vi "loadSingleToneRampData.vi"(8 "error in (no error)":errorcluster, 10 "toneRamp":refnum<class "SingleToneRamp.lvclass">, 11 "SingleToneRampAction in":refnum<class "SingleToneRampAction.lvclass">) -> (0 "error out":errorcluster, 2 "toneRampOut":refnum<class "SingleToneRamp.lvclass">, 3 "SingleToneRampAction out":refnum<class "SingleToneRampAction.lvclass">)   [LabVIEW 2011, in "Views.lvlib" / "ScriptEditor.lvlib" / "SingleToneRampAction.lvclass"]
uses:
  SingleToneRampAction.lvclass
  Tools/Scripting/ScriptingEvent/ScriptEvents/SingleTone/SingleToneRamp/SingleToneRamp.lvclass
  SingleToneRampAction.lvclass/SingleToneRampAction.ctl
  Tools/Scripting/ScriptingEvent/ScriptEvents/SingleTone/SingleTone.lvclass
  Tools/Scripting/ScriptingEvent/ScriptEvent.lvclass
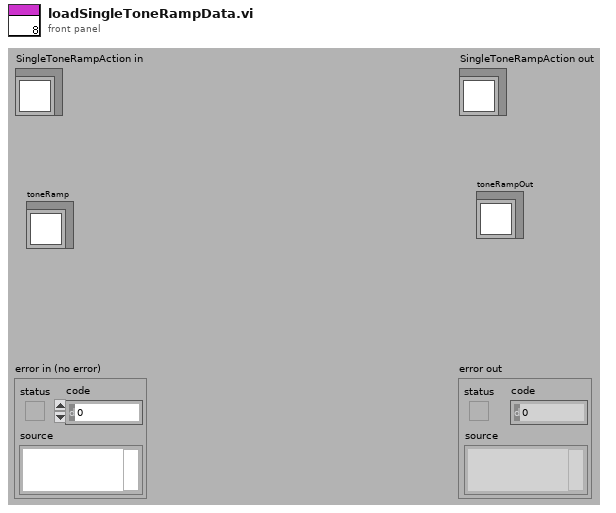
[diagram p1: front panel]
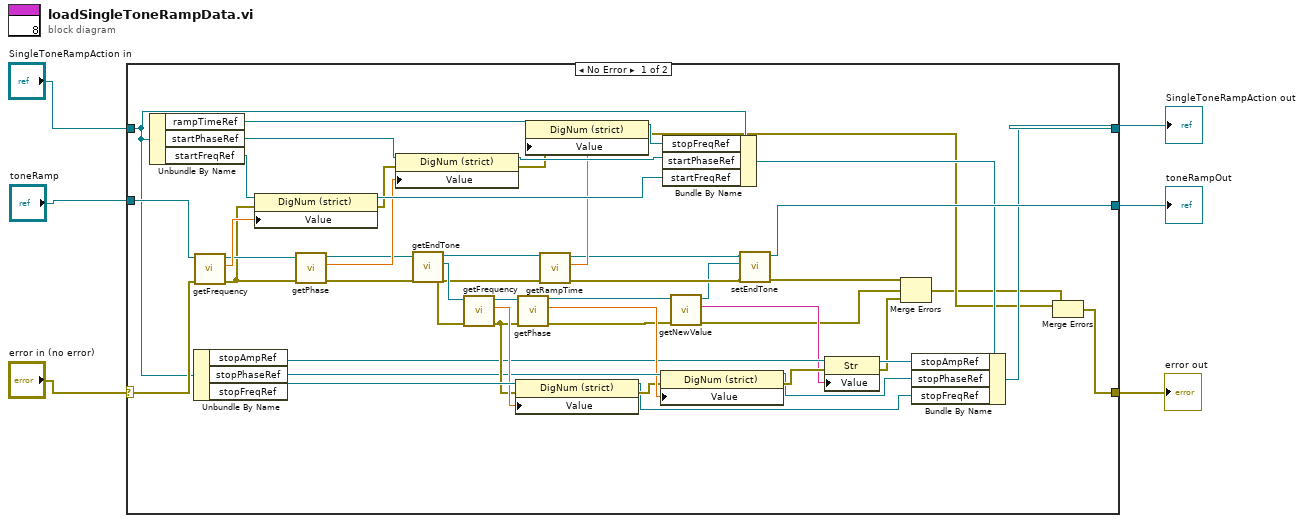
[diagram p0: block diagram]
diagram:
  n1 = case shown="No Error" "error in (no error)" {
    selector: "error in (no error)" -> [w54 w56]
    tunnel: [w12 w56] -> w2
    tunnel: [w13 w55] -> w3
    tunnel: "SingleToneRampAction in" -> [w38 w55]
    tunnel: "toneRamp" -> [w43 _]
    tunnel: [w18 _] -> w1
    frame No Error {
      n2 = Unbundle By Name(w38) -> ("rampTimeRef"=w46:refnum<vi>, "startPhaseRef"=w50:refnum<vi>, "startFreqRef"=w53:refnum<vi>)
      n3 = Unbundle By Name(w38) -> ("stopAmpRef"=w24:refnum<vi>, "stopPhaseRef"=w30:refnum<vi>, "stopFreqRef"=w37:refnum<vi>)
      n4 = call "getFrequency.vi"("error in (no error)"=w54, "SingleTone.lvclass in"=w43) -> ("error out"=w42:errorcluster, "frequency"=w52:dbl, "SingleTone.lvclass out"=w48:refnum<class "SingleToneRamp.lvclass">)  [unwired: 7 in]
      n5 = property class="DigNum (strict)"(reference=w53, error in=w42, "Value"=w52) -> (reference out=w51:refnum<vi>, error out=w41:errorcluster)
      n6 = call "getPhase.vi"("error in (no error)"=w42, "SingleTone.lvclass in"=w48) -> ("error out"=w35:errorcluster, "phase"=w44:dbl, "SingleTone.lvclass out"=w36:refnum<class "SingleToneRamp.lvclass">)  [unwired: 7 in]
      n7 = property class="DigNum (strict)"(reference=w50, error in=w41, "Value"=w44) -> (reference out=w49:refnum<vi>, error out=w47:errorcluster)
      n8 = call "getEndTone.vi"("error in (no error)"=w35, "SingleToneRamp.lvclass in"=w36) -> ("error out"=w33:errorcluster, "endTone"=w39:refnum<class "SingleTone.lvclass">, "SingleToneRamp.lvclass out"=w34:refnum<class "SingleToneRamp.lvclass">)  [unwired: 7 in]
      n9 = call "getFrequency.vi"("error in (no error)"=w33, "SingleTone.lvclass in"=w39) -> ("error out"=w31:errorcluster, "frequency"=w32:dbl, "SingleTone.lvclass out"=w28:refnum<class "SingleTone.lvclass">)  [unwired: 7 in]
      n10 = property class="DigNum (strict)"(reference=w37, error in=w31, "Value"=w32) -> (reference out=w15:refnum<vi>, error out=w25:errorcluster)
      n11 = call "getPhase.vi"("error in (no error)"=w31, "SingleTone.lvclass in"=w28) -> ("error out"=w26:errorcluster, "phase"=w29:dbl, "SingleTone.lvclass out"=w27:refnum<class "SingleTone.lvclass">)  [unwired: 7 in]
      n12 = call "getRampTime.vi"("error in (no error)"=w33, "SingleToneRamp.lvclass in"=w34) -> ("error out"=w20:errorcluster, "rampTime"=w40:dbl, "SingleToneRamp.lvclass out"=w21:refnum<class "SingleToneRamp.lvclass">)  [unwired: 7 in]
      n13 = property class="DigNum (strict)"(reference=w46, error in=w47, "Value"=w40) -> (reference out=w45:refnum<vi>, error out=w8:errorcluster)
      n14 = property class="DigNum (strict)"(reference=w30, error in=w25, "Value"=w29) -> (reference out=w16:refnum<vi>, error out=w23:errorcluster)
      n15 = Bundle By Name(cluster=w38, "stopFreqRef"=w45, "startPhaseRef"=w49, "startFreqRef"=w51) -> (w14:refnum<class "SingleToneRampAction.lvclass">)
      n16 = call "getNewValue.vi"("error in (no error)"=w26, "ScriptEvent.lvclass in"=w27) -> ("error out"=w10:errorcluster, "newValue"=w22:string, "ScriptEvent.lvclass out"=w19:refnum<class "SingleTone.lvclass">)  [unwired: 7 in]
      n17 = call "setEndTone.vi"("error in (no error)"=w20, "EndTone"=w19, "SingleToneRamp.lvclass in"=w21) -> ("error out"=w11:errorcluster, "SingleToneRamp.lvclass out"=w18:refnum<class "SingleToneRamp.lvclass">)  [unwired: 7 in]
      n18 = property class="Str"(reference=w24, error in=w23, "Value"=w22) -> (reference out=w17:refnum<vi>, error out=w9:errorcluster)
      n19 = Merge Errors(w11, w10, w9) -> (w7:errorcluster)
      n20 = Bundle By Name(cluster=w14, "stopAmpRef"=w17, "stopPhaseRef"=w16, "stopFreqRef"=w15) -> (w13:refnum<class "SingleToneRampAction.lvclass">)
      n21 = Merge Errors(w8, w7) -> (w12:errorcluster)
    }
    frame Error {
    }
  }
  "error out" <- w2
  "SingleToneRampAction out" <- w3
  "toneRampOut" <- w1
